vi "inside circle.vi"(7 "r":dbl, 8 "yc":dbl, 9 "xc":dbl, 10 "ycoords":dbl[](array[numeric]), 11 "xcoords":dbl[](array[numeric])) -> (3 "inside circle":bool[](array[boolean]))   [LabVIEW 2010]
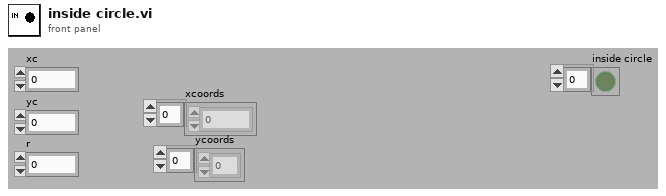
[diagram p1: front panel]
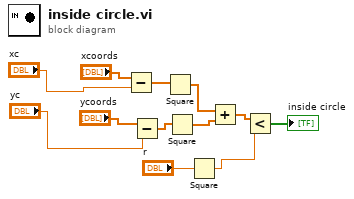
[diagram p0: block diagram]
diagram:
  n1 = Subtract(x="xcoords", y="xc") -> (x-y=w10:dbl[])
  n2 = Subtract(x="ycoords", y="yc") -> (x-y=w9:dbl[])
  n3 = Square(x=w10) -> (x^2=w8:dbl[])
  n4 = Square(x=w9) -> (x^2=w7:dbl[])
  n5 = Square(x="r") -> (x^2=w2:dbl)
  n6 = Add(x=w8, y=w7) -> (x+y=w6:dbl[])
  n7 = Less?(x=w6, y=w2) -> (x < y?=→"inside circle":bool[])
